vi "TestConvertLabviewDataRefrenceToNetObj.vi"() -> ()   [LabVIEW 2017]
panel:
  in  "milliseconds to wait":u32
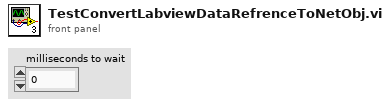
[diagram p1: front panel]
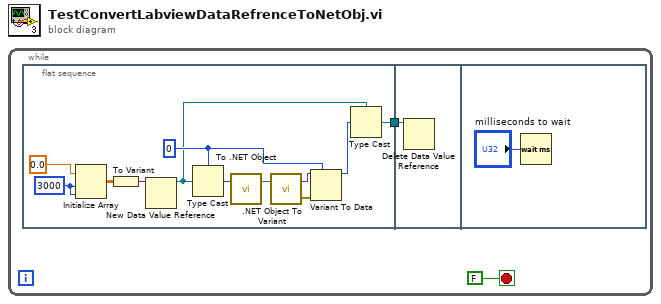
[diagram p0: block diagram]
diagram:
  n1 = while {
    stop <- FALSE stop-if-true
    n2 = flat-sequence {
      tunnel: [w3] -> w2
      tunnel: w2 -> [w15]
      frame #0 {
        w6 = u32 0
        w13 = 3000
        n3 = Initialize Array(0.0 ("element"), w13, w13) -> (w10:dbl[][])
        n4 = To Variant(anything=w10) -> (Variant=w9:variant)
        n5 = New Data Value Reference(data value=w9) -> (data value reference=w5:refnum<data-value>)  [unwired: 1 in, 1 out]
        n6 = Type Cast(type=w6, x=w5) -> (*(type *) &x=w11:u32)
        n7 = call <vilib>:"To .NET Object.vi"("anything"=w11) -> (".NET object"=w12:refnum<k24>)  [unwired: 1 in, 1 out]
        n8 = call <vilib>:".NET Object To Variant.vi"(".NET object"=w12) -> ("error out"=w8:errorcluster, "variant"=w7:variant)  [unwired: 1 in]
        n9 = Variant To Data(error in=w8, type=w6, Variant=w7) -> (data=w4:u32)  [unwired: 1 out]
        n10 = Type Cast(type=w5, x=w4) -> (*(type *) &x=w3:refnum<data-value>)
      }
      frame #1 {
        n11 = Delete Data Value Reference(data value reference=w15) -> ()  [unwired: 1 in, 2 out]
      }
      frame #2 {
        n12 = Wait (ms)(milliseconds to wait="milliseconds to wait") -> ()  [unwired: 1 out]
      }
    }
  }
